vi "NOx MFR PID loff.vi"(8 "PID gains HC":T1={"proportional gain (Kc)"=1.0, "integral time (Ti, min)"=0.1, "derivative time (Td, min)"=0.0}, 10 "NOx Up Meas":dbl format="%.2f", 11 "NOx Up SP":dbl format="%.2f") -> (2 "NO l/min":dbl)   [LabVIEW 2011]
uses:
  <vilib>/addons/control/pid/pid.llb/PID (DBL).vi
  <vilib>/addons/control/pid/NI_PID_pid.lvlib
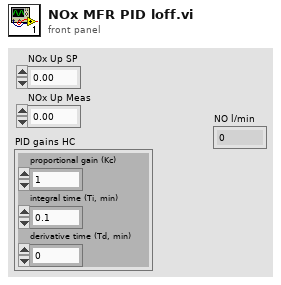
[diagram p1: front panel]
types:
  T1 = cluster{"proportional gain (Kc)":dbl, "integral time (Ti, min)":dbl, "derivative time (Td, min)":dbl}
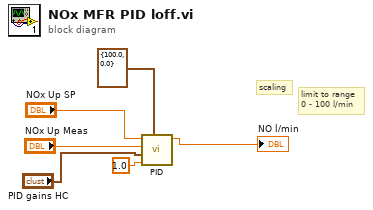
[diagram p0: block diagram]
diagram:
  # "limit to range\n0 - 100 l/min"
  # "scaling"
  n1 = call-poly <vilib>:"PID.vi"("output range"=cluster{"output high":dbl, "output low":dbl} {"output high"=100.0, "output low"=0.0}, "dt (s)"=1.0, "PID gains"="PID gains HC", "process variable"="NOx Up Meas", "setpoint"="NOx Up SP") -> ("output"=→"NO l/min":dbl)  [unwired: 5 in, 1 out]
